vi "Main_(FPGA).vi"() -> ()   [LabVIEW 2016]
uses:
  <vilib>/Platform/TimedLoop/XDataNode/timing_clust.ctl
  <vilib>/Platform/TimedLoop/XDataNode/nitl_modes.ctl
  <vilib>/Platform/TimedLoop/XDataNode/wakeup.ctl
  <vilib>/rvi/Emulation/niFpgaGetClockAttributes.vi
  <vilib>/rvi/Emulation/niFpgaSctlEmulationGetInTimedLoop.vi
  <vilib>/rvi/Emulation/niFpgaEmulationReportErrorSimple.vi
  <vilib>/rvi/Emulation/niFpgaProcessEmulError.vi
  <vilib>/rvi/Emulation/niFpgaCriticalErrorInLSC.vi
  <vilib>/rvi/eio/common/nirviEmuTemplateMethod_errors.vi
  <vilib>/rvi/interface/RandomDataEmulation/niFpgaRandomDataHandleErrors.vi
  <vilib>/eio/EIONode/EIONode.xnode
  <vilib>/rvi/DataTransferAndStorage/Container/XNode/niFpgaContainer.xnode
  <vilib>/rvi/interface/RandomDataEmulation/nirviRandomDataFpgaReadWriteTemplate.vi
  <vilib>/Platform/TimedLoop/XDataNode/XDataNode.xnode
  <vilib>/Platform/TimedLoop/XDataNode/XDNodeRunTimeDep.lvlib
panel:
  out "FPGA\nError Out":errorcluster
  out "AI0":i16
  out "Timed Out?":bool
  in  "Loop Rate (uS)":u32
  in  "FPGA I/O In  Heater (Control On/Off)":refnum<k21>="Heater_Control"
  in  "Heater Control On/Off":bool
  out "Flowrate: Period":u32
  out "Flowrate: Count":u32
  in  "Sample":bool
  out "0 = Device Present / 1=no":bool
  out "FishtankTemperature (raw)":u16
  out "Scratchpad Data":u8[](array[numeric])
  out "error out":errorcluster
  in  "FPGA I/O In (Control On/Off) 2":refnum<k21>="Pump_Control"
  in  "Pump Control On/Off":bool
  in  "FPGA I/O Out (Trigger Pulse) 2":refnum<k21>="UTR1_Trigger"
  in  "FPGA I/O In (Echo) 2":refnum<k21>="UTR1_Echo"
  out "Measured Period (usec) - Growbed":u32
  out "Input Signal (Out) 2":bool
  in  "Low Pulse (usec) 2":u32=100000
  in  "High Pulse(usec) 2":u32=5
  out "Output Pulse 2":bool
  in  "FPGA I/O In (Control On/Off)":refnum<k21>="Add_Water_Control"
  in  "Add Water Control On/Off":bool
  in  "FPGA I/O Out (Trigger Pulse)":refnum<k21>="UTR2_Trigger"
  in  "FPGA I/O In (Echo)":refnum<k21>="UTR2_Echo"
  out "Measured Period (usec) - Fishtank":u32
  out "Input Signal (Out)":bool
  in  "Low Pulse (usec)":u32=100000
  in  "High Pulse(usec)":u32=5
  out "Output Pulse":bool
  in  "stop":bool
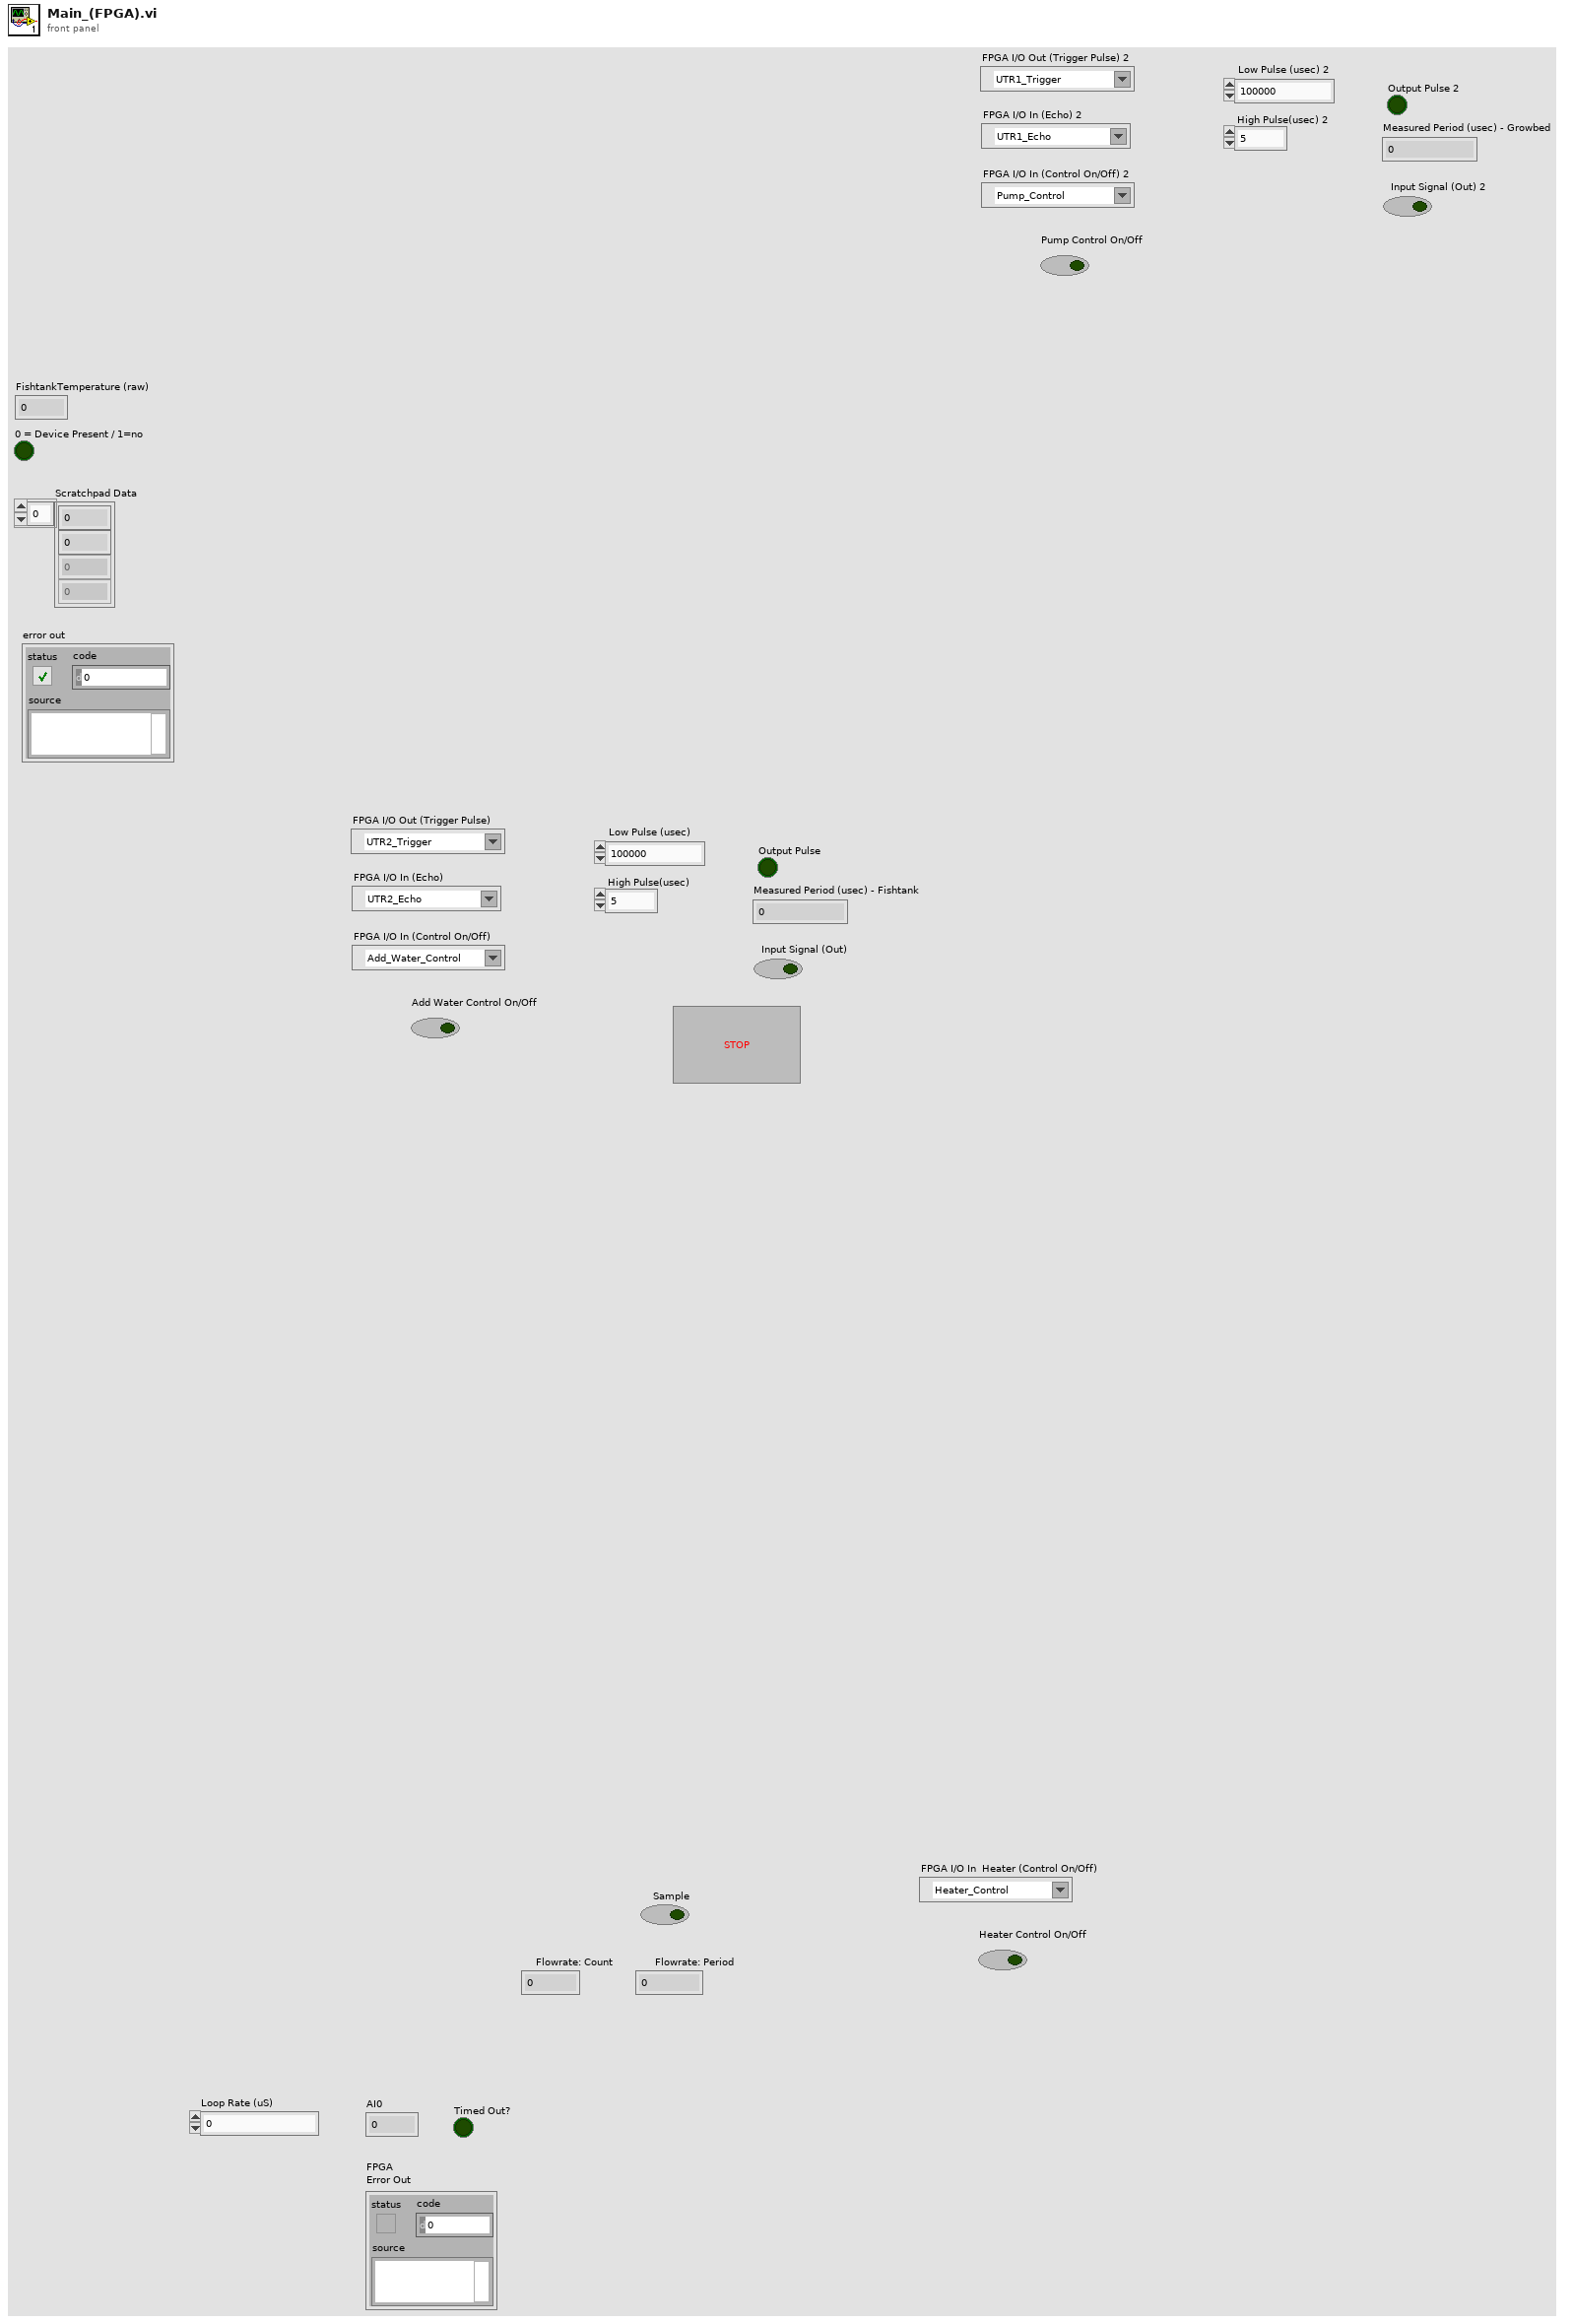
[diagram p1: front panel]
types:
  T1 = typedef "XDNodeRunTimeDep.lvlib/timing_clust.ctl" = cluster{"Expected End [f-1]":u64, "Actual End [f-1]":u64, "Finished Late? [f-1]":bool, "Expected End [i-1]":u64, "Actual End [i-1]":u64, "Finished Late? [i-1]":bool, "Expected Start [i]":u64, "Actual Start [i]":u64, "Expected Start [f]":u64, "Actual Start [f]":u64, "Source Name":string, "Structure Name":string, "Period":i64, "Deadline":i64, "Offset":i64, "Start":i64, "Priority":i32, "Timeout":i32, "Mode":T2, "Wakeup Reason":T3, "Error":errorcluster, "Source Type":string, "Secondary Source Type":string, "Global End Time":u64, "Global Start Time":u64, "Frame Duration":u64, "Iteration Duration":u64, "Assigned CPU":i32, "I/O Scan Engine Mode":u32}
  T2 = typedef "XDNodeRunTimeDep.lvlib/nitl_modes.ctl" = enum32{"No Change", "Process missed periods, maintain original phase", "Discard missed periods, maintain original phase", "Process missed periods, ignore original phase", "Discard missed periods, ignore original phase"}
  T3 = typedef "XDNodeRunTimeDep.lvlib/wakeup.ctl" = enum32{"Normal", "Aborted", "Asynchronous wakeup", "Timing source error", "Timed loop error", "Timeout"}
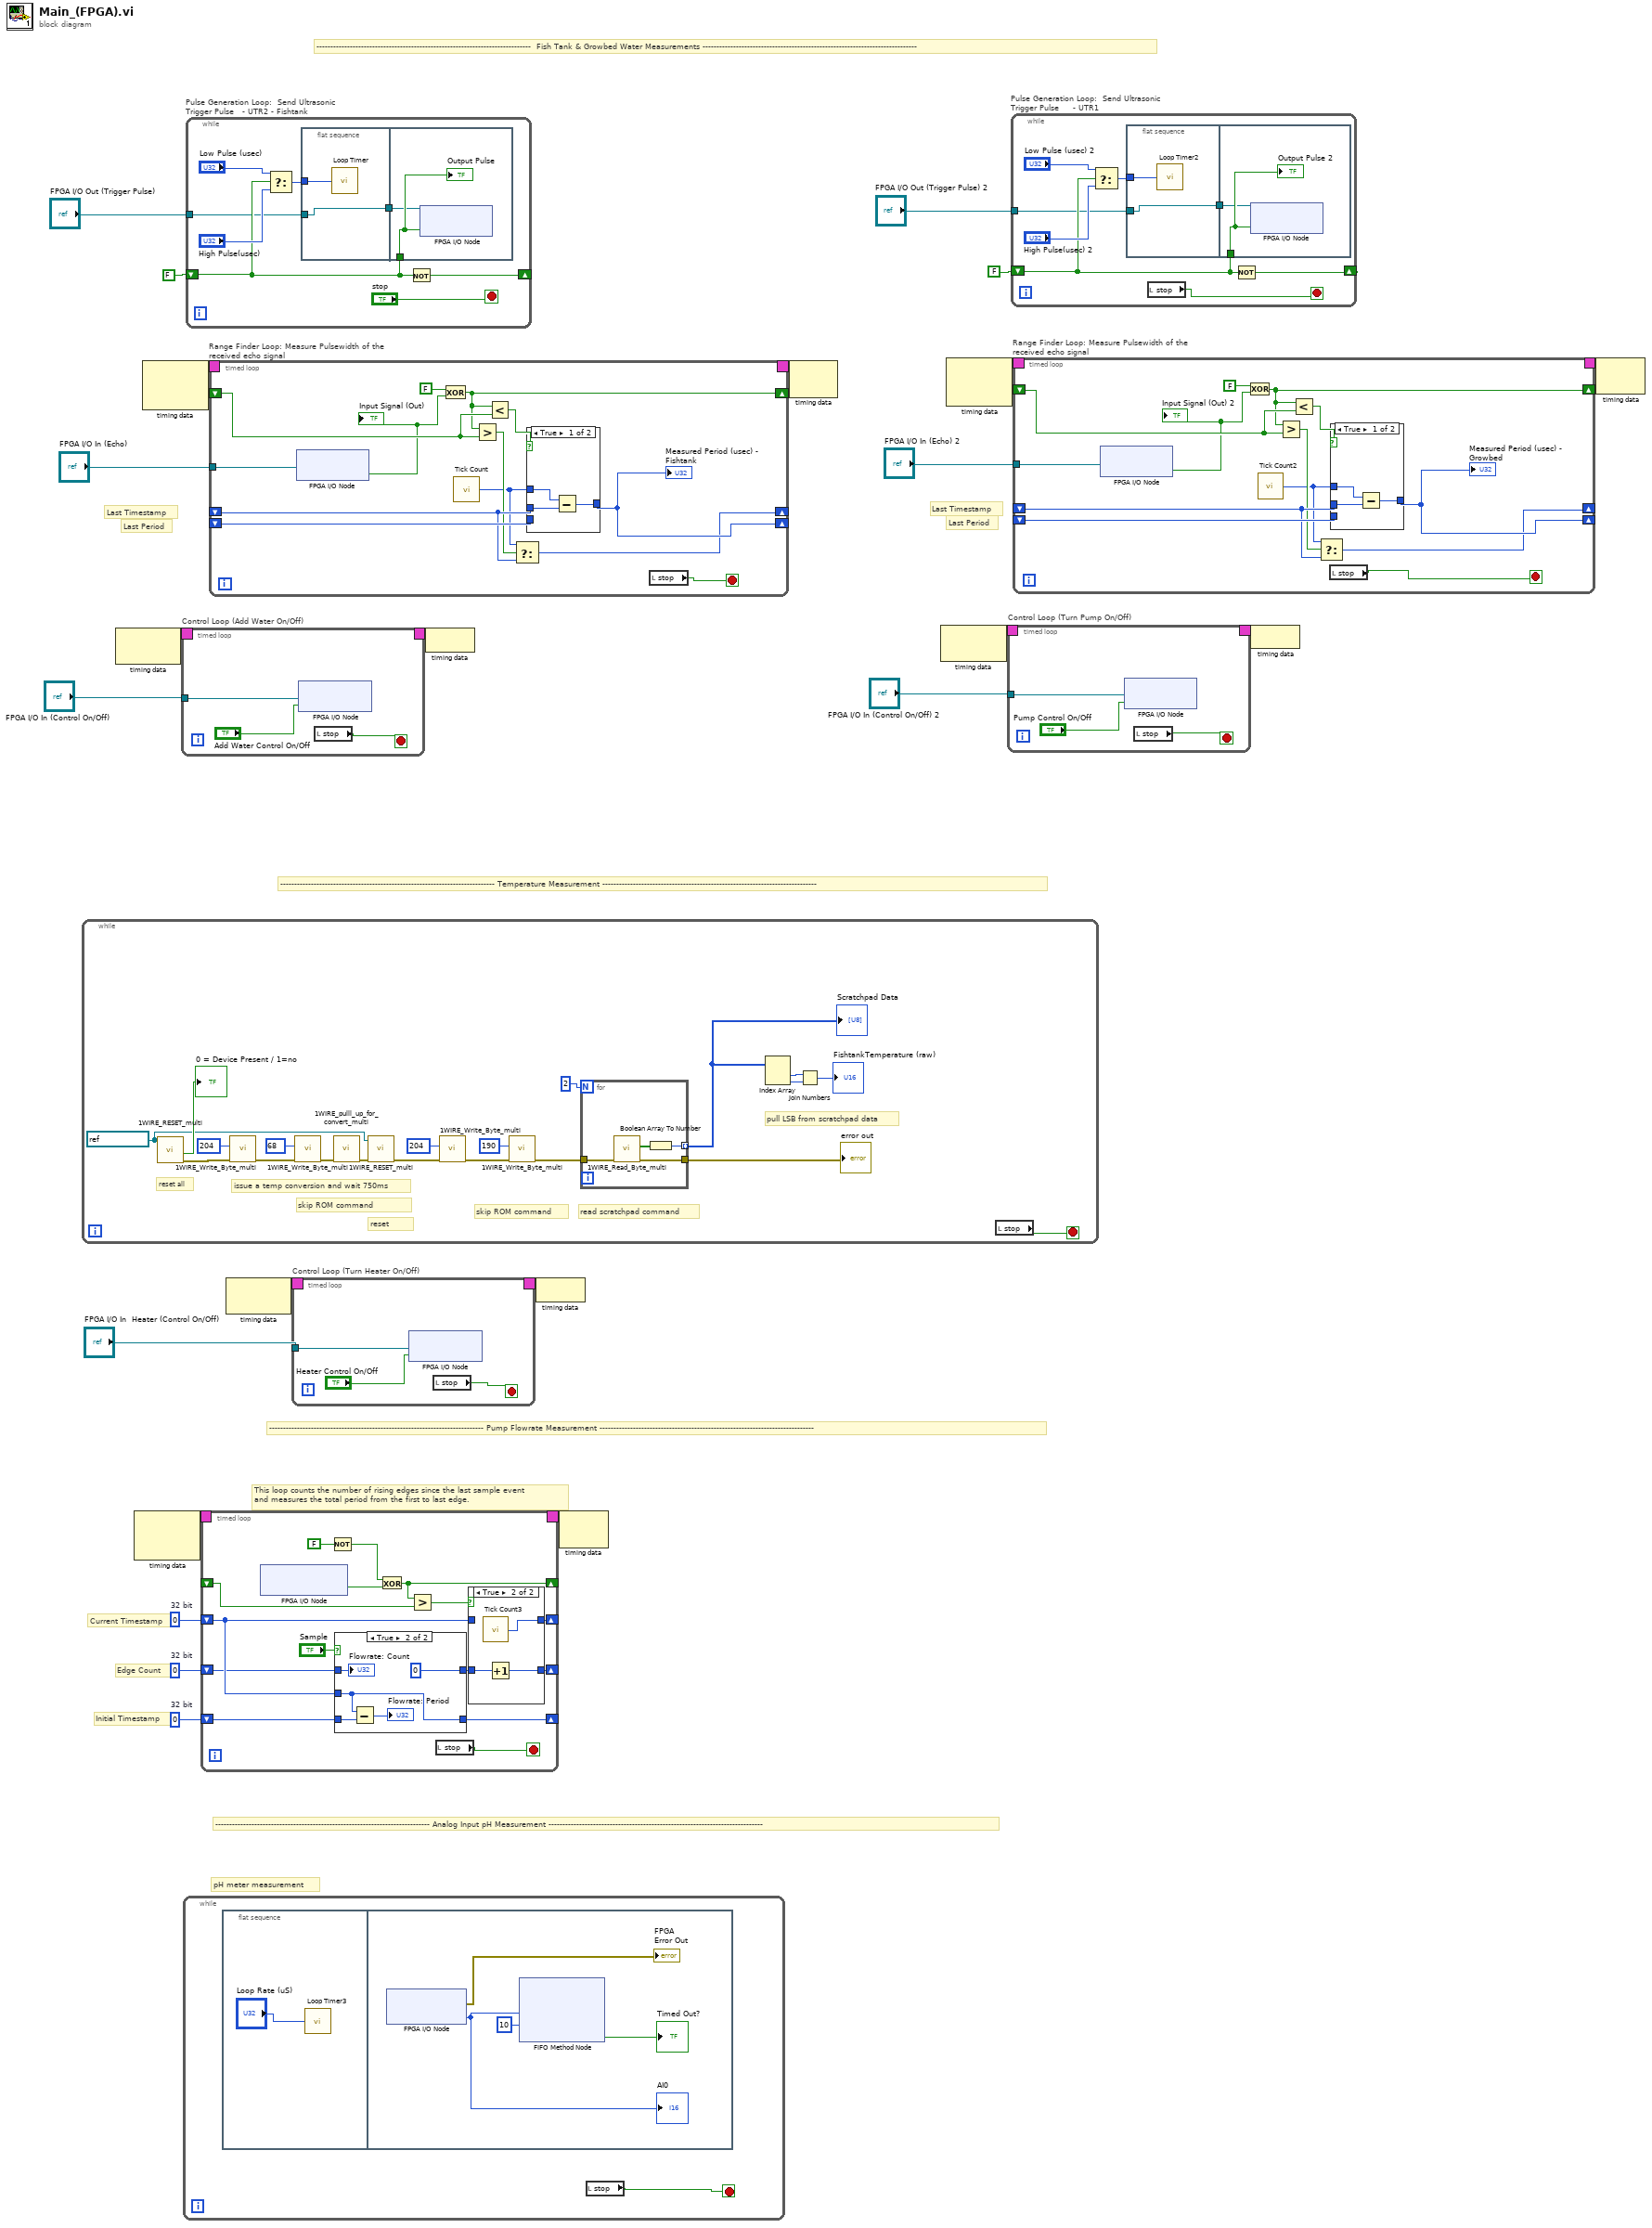
[diagram p0: block diagram]
diagram:
  w5 = u32 0  # 32 bit
  w4 = u32 0  # 32 bit
  w6 = u32 0  # 32 bit
  # "pH meter measurement"
  # "----------------------------------------------------------------------------- Analog Input pH Measurement -----------------------------------------------------------------------------"
  # "----------------------------------------------------------------------------- Pump Flowrate Measurement -----------------------------------------------------------------------------"
  # "This loop counts the number of rising edges since the last sample event\nand measures the total period from the first to last edge."
  # "Initial Timestamp"
  # "Edge Count"
  # "Current Timestamp"
  # "-----------------------------------------------------------------------------  Fish Tank & Growbed Water Measurements -----------------------------------------------------------------------------"
  # "----------------------------------------------------------------------------- Temperature Measurement -----------------------------------------------------------------------------"
  # "Last Period"
  # "Last Timestamp"
  # "Last Period"
  # "Last Timestamp"
  n1 = while {
    stop <- w25 stop-if-true
    w26 = refnum<k21> "DS_WIRE" ("FPGA I/O In")
    # "pull LSB from scratchpad data"
    # "read scratchpad command"
    # "skip ROM command"
    # "reset"
    # "issue a temp conversion and wait 750ms"
    # "skip ROM command"
    # "reset all"
    n2 = call "1WIRE_RESET_multi.vi"("FPGA I/O In"=w26) -> ("error out"=w31:errorcluster, "0 = Device Present / 1=no"=→"0 = Device Present / 1=no":bool)  [unwired: 9 in]
    n3 = call "1WIRE_Write_Byte_multi.vi"("error in"=w31, "Tx data"=u8 204 ("Tx data 2")) -> ("error out"=w30:errorcluster)  [unwired: 8 in, 1 out]
    n4 = call "1WIRE_Write_Byte_multi.vi"("error in"=w30, "Tx data"=u8 68 ("Tx data 2")) -> ("error out"=w43:errorcluster)  [unwired: 8 in, 1 out]
    n5 = call "1WIRE_pulll_up_for_convert_multi.vi"("error in"=w43) -> ("error out"=w32:errorcluster)  [unwired: 10 in]
    n6 = call "1WIRE_RESET_multi.vi"("error in"=w32, "FPGA I/O In"=w26) -> ("error out"=w33:errorcluster)  [unwired: 8 in, 1 out]
    n7 = call "1WIRE_Write_Byte_multi.vi"("error in"=w33, "Tx data"=u8 204 ("Tx data 2")) -> ("error out"=w34:errorcluster)  [unwired: 8 in, 1 out]
    n8 = call "1WIRE_Write_Byte_multi.vi"("error in"=w34, "Tx data"=u8 190 ("Tx data 2")) -> ("error out"=w36:errorcluster)  [unwired: 8 in, 1 out]
    n9 = for {
      N: 2 -> [_]
      tunnel: w36 -> [w48]
      tunnel: [w47] -> w27
      tunnel: [w46] -> w39 mode=indexing
      n10 = call "1WIRE_Read_Byte_multi.vi"("error in"=w48) -> ("error out"=w47:errorcluster, "Array"=w45:bool[])  [unwired: 9 in]
      n11 = Boolean Array To Number(Boolean array=w45) -> (number=w46:u8)
    }
    "Scratchpad Data" <- w39
    "error out" <- w27
    n12 = Index Array(array=w39) -> (element #1=w38:u8, element #2=w40:u8)  [unwired: 2 in]
    n13 = Join Numbers(hi=w38, lo=w40) -> ((hi.lo)=→"FishtankTemperature (raw)":u16)
    n14 = local read "stop"() -> (w25:bool)
  }
  n15 = node-c288() -> (w22:T1)  [unwired: 1 in]
  n16 = node-c288() -> (w8:T1)  [unwired: 2 out]
  n17 = node-c288() -> (w24:T1)  [unwired: 2 out]
  n18 = timed-loop "Control Loop (Add Water On/Off)" {
    timing: w22 -> [_]
    timing-out: [_] -> w21
    tunnel: "FPGA I/O In (Control On/Off)" -> [w51]
    stop <- w49 stop-if-true
    n19 = xnode "FPGA I/O Node"("I/O Item"="Add Water Control On/Off", "FPGA I/O In"=w51) -> ()  [unwired: 1 out]
    n20 = local read "stop"() -> (w49:bool)
  }
  n21 = while {
    stop <- w54 stop-if-true
    n22 = flat-sequence {
      frame #0 {
        n23 = call "Loop Timer3"("Count(uSec)"="Loop Rate (uS)") -> ()  [unwired: 1 out]
      }
      frame #1 {
        n24 = xnode "FPGA I/O Node"() -> ("error out"=→"FPGA\nError Out":errorcluster, "pH_Meter"=w59:i16)  [unwired: 2 in, 1 out]
        "AI0" <- w59
        n25 = xnode ("FIFO Method Node")("Element"=w59, "Timeout"=10) -> ("Timed Out?"=→"Timed Out?":bool)  [unwired: 1 in, 1 out]
      }
    }
    n26 = local read "stop"() -> (w54:bool)
  }
  n27 = while "Pulse Generation Loop:  Send Ultrasonic Trigger Pulse   - UTR2 - Fishtank" {
    shift-right: [w63] -> _
    shift-left: FALSE -> [w64]
    tunnel: "FPGA I/O Out (Trigger Pulse)" -> [w61]
    stop <- "stop" stop-if-true
    n28 = Select(t="Low Pulse (usec)", s=w64, f="High Pulse(usec)") -> (s? t:f=w65:u32)
    n29 = flat-sequence {
      tunnel: w65 -> [w69]
      tunnel: w61 -> [w68]
      tunnel: [w68] -> w60
      tunnel: w64 -> [w71]
      tunnel: w60 -> [w70]
      frame #0 {
        n30 = call "Loop Timer"("Count(uSec)"=w69) -> ()  [unwired: 1 out]
      }
      frame #1 {
        n31 = xnode "FPGA I/O Node"("I/O Item"=w71, "FPGA I/O In"=w70) -> ()  [unwired: 1 out]
        "Output Pulse" <- w71
      }
    }
    n32 = Not(x=w64) -> (.not. x?=w63:bool)
  }
  n33 = timed-loop {
    timing-out: [_] -> w7
    timing: w8 -> [_]
    shift-left: w5 -> [w78]
    shift-right: [w79] -> _
    shift-left: w4 -> [w80]
    shift-right: [w82] -> _
    shift-left: w6 -> [w77]
    shift-right: [w83] -> _
    shift-left: _ -> [w85]
    shift-right: [w86] -> _
    stop <- w73 stop-if-true
    n34 = xnode "FPGA I/O Node"() -> ("Flow_meter"=w74:bool)  [unwired: 1 in, 1 out]
    n35 = Not(x=FALSE) -> (.not. x?=w75:bool)
    n36 = case shown="True" "Sample" {
      tunnel: w80 -> [_ w93]
      tunnel: [w87 w93] -> w79
      tunnel: w78 -> [w87 w92]
      tunnel: w77 -> [w88 w90]
      tunnel: [w88 u32 0 ("32 bit")] -> w76
      frame False {
      }
      frame True {
        n37 = Subtract(x=w93, y=w92) -> (x-y=→"Flowrate: Period":u32)
        "Flowrate: Count" <- w90
      }
    }
    n38 = Exclusive Or(1:w74, 2:w75) -> (0:w86:bool)
    n39 = Greater?(x=w86, y=w85) -> (0:w84:bool)
    n40 = local read "stop"() -> (w73:bool)
    n41 = case shown="True" w84 {
      tunnel: w76 -> [w94 w98]
      tunnel: [w94 w97] -> w83
      tunnel: [w95 w96] -> w82
      tunnel: w80 -> [w95 _]
      frame False {
      }
      frame True {
        n42 = call "Tick Count3"() -> ("Tick Count(Ticks)"=w96:u32)
        n43 = Increment(x=w98) -> (x+1=w97:u32)
      }
    }
  }
  n44 = timed-loop "Range Finder Loop: Measure Pulsewidth of the received echo signal" {
    timing-out: [_] -> w23
    timing: w24 -> [_]
    shift-left: _ -> [w112]
    shift-right: [w113] -> _
    shift-left: _ -> [w111]
    shift-right: [w110] -> _
    shift-left: _ -> [w108]
    shift-right: [w106] -> _
    tunnel: "FPGA I/O In (Echo)" -> [w103]
    stop <- w102 stop-if-true
    n45 = xnode "FPGA I/O Node"("FPGA I/O In"=w103) -> ("I/O Item"=w104:bool)  [unwired: 1 out]
    "Input Signal (Out)" <- w104
    n46 = Exclusive Or(1:w104, 2:FALSE ("x")) -> (0:w106:bool)
    n47 = call "Tick Count"() -> ("Tick Count(uSec)"=w105:u32)
    n48 = Greater?(x=w106, y=w108) -> (0:w109:bool)
    n49 = Less?(x=w106, y=w108) -> (x < y?=w107:bool)
    n50 = Select(t=w105, s=w109, f=w111) -> (s? t:f=w110:u32)
    n51 = case shown="True" w107 {
      tunnel: w112 -> [_ w117]
      tunnel: w105 -> [w114 _]
      tunnel: w111 -> [w115 _]
      tunnel: [w116 w117] -> w113
      frame True {
        n52 = Subtract(x=w114, y=w115) -> (x-y=w116:u32)
      }
      frame False {
      }
    }
    "Measured Period (usec) - Fishtank" <- w113
    n53 = local read "stop"() -> (w102:bool)
  }
  n54 = node-c288() -> (w3:T1)  [unwired: 1 in]
  n55 = timed-loop "Control Loop (Turn Heater On/Off)" {
    timing: w3 -> [_]
    timing-out: [_] -> w2
    tunnel: "FPGA I/O In  Heater (Control On/Off)" -> [w122]
    stop <- w120 stop-if-true
    n56 = xnode "FPGA I/O Node"("I/O Item"="Heater Control On/Off", "FPGA I/O In"=w122) -> ()  [unwired: 1 out]
    n57 = local read "stop"() -> (w120:bool)
  }
  n58 = node-c288(w21) -> ()
  n59 = node-c288(w2) -> ()
  n60 = node-c288(w7) -> ()  [unwired: 1 out]
  n61 = node-c288(w23) -> ()  [unwired: 1 out]
  n62 = node-c288() -> (w14:T1)  [unwired: 1 in]
  n63 = node-c288() -> (w16:T1)  [unwired: 2 out]
  n64 = timed-loop "Control Loop (Turn Pump On/Off)" {
    timing: w14 -> [_]
    timing-out: [_] -> w13
    tunnel: "FPGA I/O In (Control On/Off) 2" -> [w127]
    stop <- w125 stop-if-true
    n65 = xnode "FPGA I/O Node"("I/O Item"="Pump Control On/Off", "FPGA I/O In"=w127) -> ()  [unwired: 1 out]
    n66 = local read "stop"() -> (w125:bool)
  }
  n67 = while "Pulse Generation Loop:  Send Ultrasonic Trigger Pulse     - UTR1" {
    shift-right: [w133] -> _
    shift-left: FALSE -> [w134]
    tunnel: "FPGA I/O Out (Trigger Pulse) 2" -> [w132]
    stop <- w130 stop-if-true
    n68 = Select(t="Low Pulse (usec) 2", s=w134, f="High Pulse(usec) 2") -> (s? t:f=w135:u32)
    n69 = flat-sequence {
      tunnel: w135 -> [w139]
      tunnel: w132 -> [w138]
      tunnel: [w138] -> w131
      tunnel: w134 -> [w141]
      tunnel: w131 -> [w140]
      frame #0 {
        n70 = call "Loop Timer2"("Count(uSec)"=w139) -> ()  [unwired: 1 out]
      }
      frame #1 {
        n71 = xnode "FPGA I/O Node"("I/O Item"=w141, "FPGA I/O In"=w140) -> ()  [unwired: 1 out]
        "Output Pulse 2" <- w141
      }
    }
    n72 = local read "stop"() -> (w130:bool)
    n73 = Not(x=w134) -> (.not. x?=w133:bool)
  }
  n74 = timed-loop "Range Finder Loop: Measure Pulsewidth of the received echo signal" {
    timing-out: [_] -> w15
    timing: w16 -> [_]
    shift-left: _ -> [w153]
    shift-right: [w154] -> _
    shift-left: _ -> [w152]
    shift-right: [w151] -> _
    shift-left: _ -> [w149]
    shift-right: [w147] -> _
    tunnel: "FPGA I/O In (Echo) 2" -> [w144]
    stop <- w143 stop-if-true
    n75 = xnode "FPGA I/O Node"("FPGA I/O In"=w144) -> ("I/O Item"=w145:bool)  [unwired: 1 out]
    "Input Signal (Out) 2" <- w145
    n76 = Exclusive Or(1:w145, 2:FALSE ("x")) -> (0:w147:bool)
    n77 = call "Tick Count2"() -> ("Tick Count(uSec)"=w146:u32)
    n78 = Greater?(x=w147, y=w149) -> (0:w150:bool)
    n79 = Less?(x=w147, y=w149) -> (x < y?=w148:bool)
    n80 = Select(t=w146, s=w150, f=w152) -> (s? t:f=w151:u32)
    n81 = local read "stop"() -> (w143:bool)
    n82 = case shown="True" w148 {
      tunnel: w153 -> [_ w158]
      tunnel: w146 -> [w155 _]
      tunnel: w152 -> [w156 _]
      tunnel: [w157 w158] -> w154
      frame True {
        n83 = Subtract(x=w155, y=w156) -> (x-y=w157:u32)
      }
      frame False {
      }
    }
    "Measured Period (usec) - Growbed" <- w154
  }
  n84 = node-c288(w13) -> ()
  n85 = node-c288(w15) -> ()  [unwired: 1 out]
